vi "Read data.vi"(11 "LinealFitting in":refnum<class "LinealFitting.lvclass">) -> (0 "residue":dbl, 2 "slope":dbl)   [LabVIEW 2019, in "LinealFitting.lvclass"]
uses:
  LinealFitting.lvclass
  LinealFitting.lvclass/LinealFitting.ctl
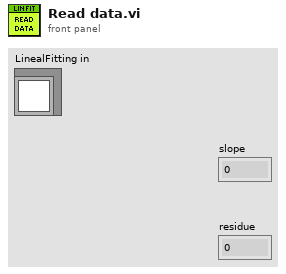
[diagram p1: front panel]
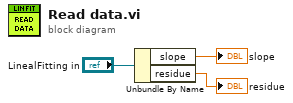
[diagram p0: block diagram]
diagram:
  n1 = Unbundle By Name("LinealFitting in") -> ("slope"=→"slope":dbl, "residue"=→"residue":dbl)
